vi "Response Message.vi"(8 "error in (no error)":errorcluster, 9 "Response Message Data":variant, 10 "Response Message":string, 11 "Process In":refnum<class "Debug View.lvclass">) -> (0 "error out":errorcluster, 3 "Process Out":refnum<class "Debug View.lvclass">)   [LabVIEW 2020]
doc: "Respond to a request message. The response will only be delivered to the requesting method and. \nThis VI may only be called from within the same case of the Handle Messages VI which handles the request or from a Helper Loop or Asynchronous Action launched from the specific case."
uses:
  Debug View.lvclass
  Debug View.lvclass/Debug View.ctl
  Request Message Cluster.ctl
  <vilib>/Utility/error.llb/Clear Errors.vi
  <vilib>/Utility/error.llb/Error Cluster From Error Code.vi
  <vilib>/ErrorRing/Error Ring.xnode
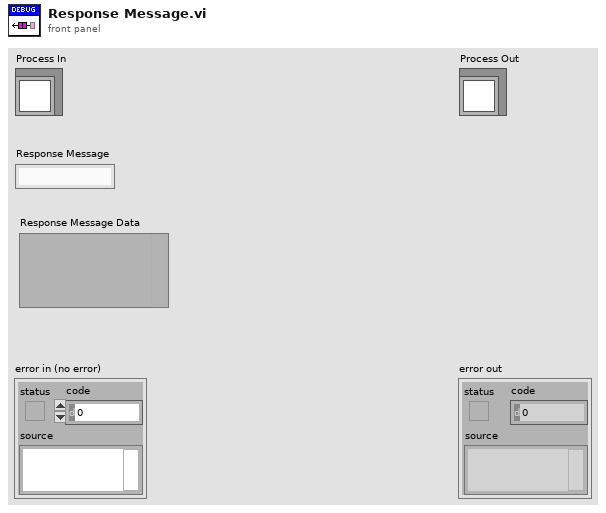
[diagram p1: front panel]
types:
  T1 = typedef "Lifecycle State.ctl" = enum16{"Uninitialized", "Initialized", "Started", "Running", "Stopped", "Finished"}
  T2 = typedef "Debug View.lvclass/Request Message Cluster.ctl" = cluster{"Message":string, "Message Data":variant, "Request Error":errorcluster}
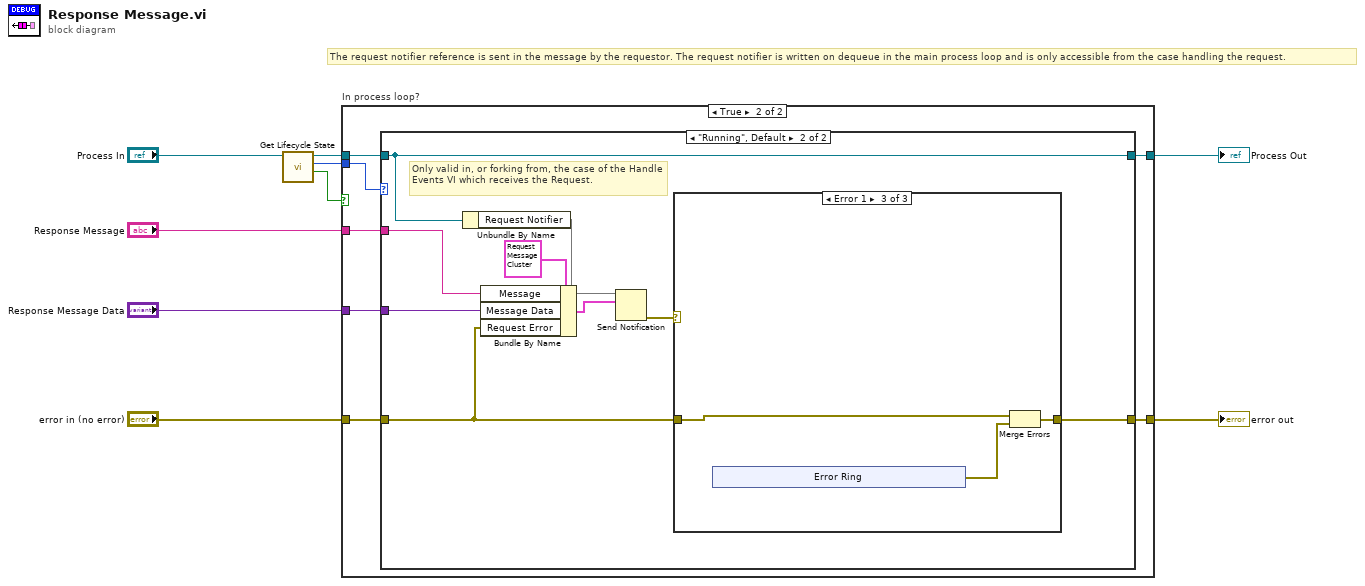
[diagram p0: block diagram]
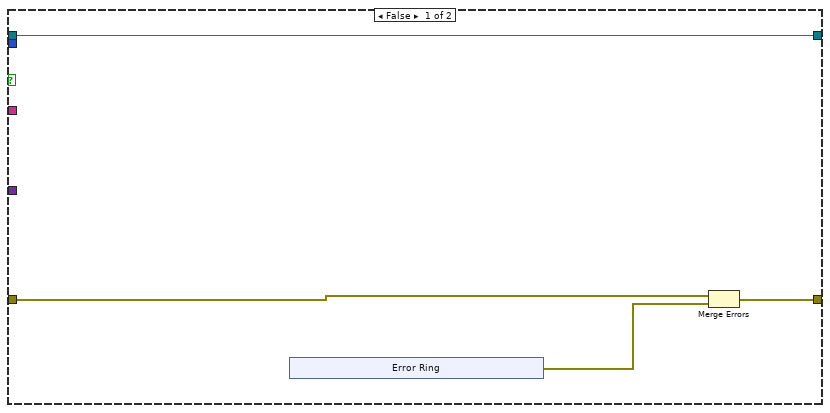
[diagram p2: hidden frame]
diagram:
  # "The request notifier reference is sent in the message by the requestor. The request notifier is written on dequeue in the main process loop and is only accessible from the case handling the request."
  n1 = call "Get Lifecycle State.vi"("Process In"="Process In") -> ("In Process Loop?"=w1:bool, "Lifecycle State"=w2:T1, "Process Out"=w3:refnum<class "Debug View.lvclass">)  [unwired: 7 in, 1 out]
  n2 = case "In process loop?" shown="True" w1 {
    tunnel: "Response Message" -> [_ w24]
    tunnel: "Response Message Data" -> [_ w23]
    tunnel: [w12 w22] -> w5
    tunnel: w3 -> [w13 w21]
    tunnel: "error in (no error)" -> [w11 w20]
    tunnel: w2 -> [_ w19]
    tunnel: [w13 w18] -> w4
    frame False {
      n3 = xnode "Error Ring"() -> ("error out"=w10:errorcluster)
      n4 = Merge Errors(w11, w10) -> (w12:errorcluster)
    }
    frame True {
      n5 = case shown="\"Running\", Default" w19 {
        tunnel: w24 -> [_ w32]
        tunnel: w23 -> [_ w31]
        tunnel: [w25 w29] -> w22
        tunnel: w21 -> [w26 w28]
        tunnel: w20 -> [w25 w27]
        tunnel: [w26 w28] -> w18
        frame "Stopped" {
          # "If the process is stopped, the wait for reply VI will abort and throw an error. \nThere is no reason to throw an error here as well."
        }
        frame "Running", Default {
          # "Only valid in, or forking from, the case of the Handle Events VI which receives the Request."
          n6 = Unbundle By Name(w28) -> ("Request Notifier"=w35)
          n7 = Bundle By Name(cluster=T2 {"Message"="", "Message Data"=variant, "Request Error"={"status"=FALSE, "code"=0, "source"=""}} ("notification"), "Message"=w32, "Message Data"=w31, "Request Error"=w27) -> (w33:T2)
          n8 = Send Notification(notification=w33, notifier=w35) -> (error out=w30:errorcluster)  [unwired: 1 in, 1 out]
          n9 = case shown="Error 1" w30 {
            selector: w30 -> [w36 w37 _]
            tunnel: [w36 w37 w39] -> w29
            tunnel: w27 -> [_ _ w38]
            frame No Error {
            }
            frame Default {
            }
            frame Error {
              n10 = xnode "Error Ring"() -> ("error out"=w40:errorcluster)
              n11 = Merge Errors(w38, w40) -> (w39:errorcluster)
            }
          }
        }
      }
    }
  }
  "error out" <- w5
  "Process Out" <- w4
